vi "Create and merge label lists.vi"(8 "error in (no error)":errorcluster, 9 "Ordered item labels":string[](array[string]), 10 "Override parent list":string[](array[string]), 11 "Override item list":string[](array[string])) -> (0 "error out":errorcluster, 2 "Merged parent list":string[](array[string]), 3 "Merged item list":string[](array[string]), 4 "ordered parents not found":string[](array[string]), 6 "ordered items not found":string[](array[string]))   [LabVIEW 2020, in "verticalDistribution.lvlib"]
uses:
  <vilib>/Utility/vertDist/verticalDistribution.lvlib
panel:
  # "If items not found\nthen they will fail\nto be aligned!"
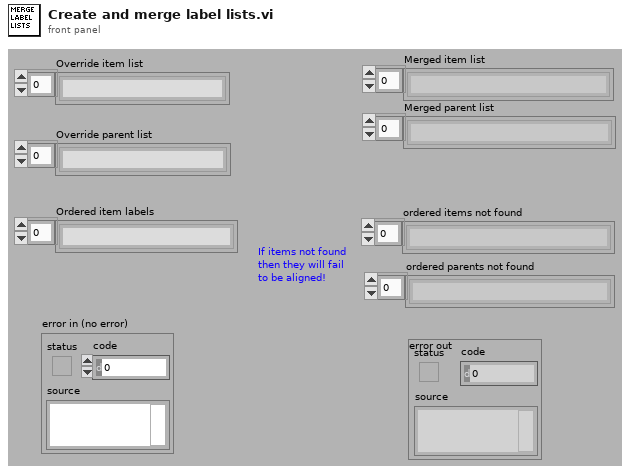
[diagram p1: front panel]
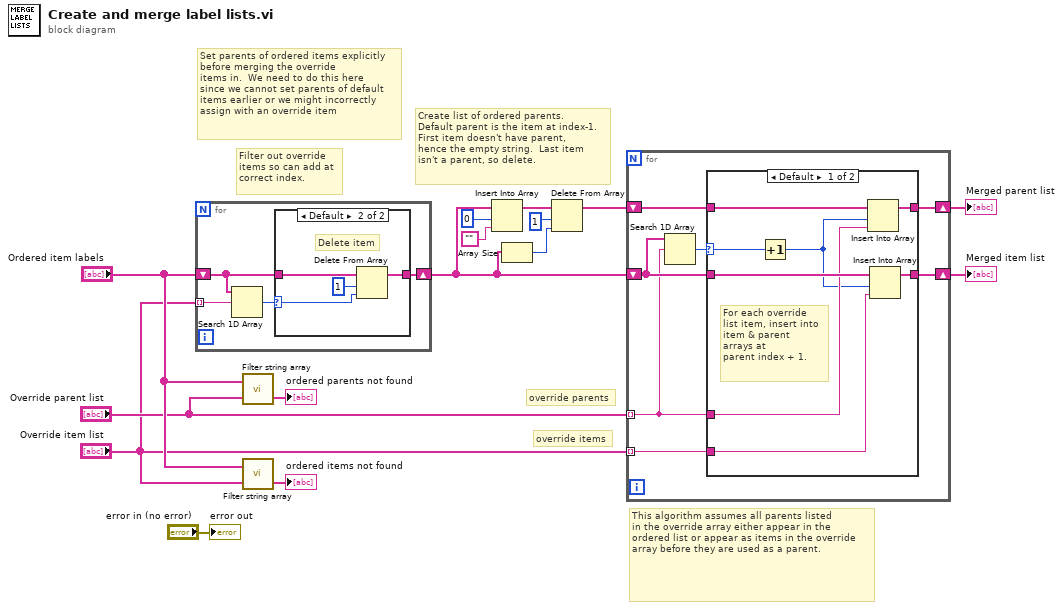
[diagram p0: block diagram]
diagram:
  # "override items"
  # "Create list of ordered parents.\nDefault parent is the item at index-1.\nFirst item doesn't have parent,\nhence the empty string.  Last item\nisn't a parent, so delete."
  # "Set parents of ordered items explicitly \nbefore merging the override\nitems in.  We need to do this here\nsince we cannot set parents of default\nitems earlier or we might incorrectly\nassign with an override item"
  # "override parents"
  # "This algorithm assumes all parents listed\nin the override array either appear in the\nordered list or appear as items in the override\narray before they are used as a parent."
  # "Filter out override\nitems so can add at\ncorrect index."
  n1 = for {
    shift-right: [w17] -> w5
    shift-left: "Ordered item labels" -> [w18]
    tunnel: "Override item list" -> [w16] mode=indexing
    n2 = Search 1D Array(1D array=w18, element=w16) -> (index of element=w19:i32)  [unwired: 1 out]
    n3 = case shown="Default" w19 {
      selector: w19 -> [_ w22]
      tunnel: w18 -> [w20 w24]
      tunnel: [w20 w23] -> w17
      frame -1 {
      }
      frame Default {
        # "Delete item"
        n4 = Delete From Array(array=w24, length=1, index=w22) -> (array with subset deleted=w23:string[])  [unwired: 1 out]
      }
    }
  }
  n5 = call <vilib>:"Filter string array.vi"("Elements to Match"="Override parent list", "Array to Search"="Ordered item labels") -> ("Remaining Elements"=→"ordered parents not found":string[])  [unwired: 1 out]
  n6 = call <vilib>:"Filter string array.vi"("Elements to Match"="Override item list", "Array to Search"="Ordered item labels") -> ("Remaining Elements"=→"ordered items not found":string[])  [unwired: 1 out]
  n7 = Insert Into Array(array=w5, index=0, new element="") -> (w7:string[])
  n8 = Array Size(array=w5) -> (size(s)=w4:i32)
  n9 = Delete From Array(array=w7, length=1, index=w4) -> (array with subset deleted=w3:string[])  [unwired: 1 out]
  n10 = for {
    tunnel: "Override item list" -> [w29] mode=indexing
    shift-right: [w30] -> w11
    shift-left: w5 -> [w31]
    tunnel: "Override parent list" -> [w25] mode=indexing
    shift-right: [w26] -> w10
    shift-left: w3 -> [w28]
    n11 = Search 1D Array(1D array=w31, element=w25) -> (index of element=w27:i32)  [unwired: 1 out]
    n12 = case shown="Default" w27 {
      selector: w27 -> [w32 _]
      tunnel: w31 -> [w37 w41]
      tunnel: [w39 w41] -> w30
      tunnel: w29 -> [w38 _]
      tunnel: w28 -> [w34 w40]
      tunnel: w25 -> [w36 _]
      tunnel: [w33 w40] -> w26
      frame Default {
        # "For each override\nlist item, insert into \nitem & parent\narrays at \nparent index + 1."
        n13 = Increment(x=w32) -> (x+1=w35:i32)
        n14 = Insert Into Array(array=w34, index=w35, new element=w36) -> (w33:string[])
        n15 = Insert Into Array(array=w37, index=w35, new element=w38) -> (w39:string[])
      }
      frame -1 {
        # "Parent of override item not found.  Skip item since we don't know what to do with it."
      }
    }
  }
  "Merged item list" <- w11
  "Merged parent list" <- w10
  "error out" <- "error in (no error)"
